vi "Health Status Screen 2.vi"() -> ()   [LabVIEW 2022 SP3]
panel:
  out "?":bool
  out "?":bool
  out "?":bool
  out "?":bool
  out "?":bool
  in  "Button":bool
  # "HEALTH STATUS"
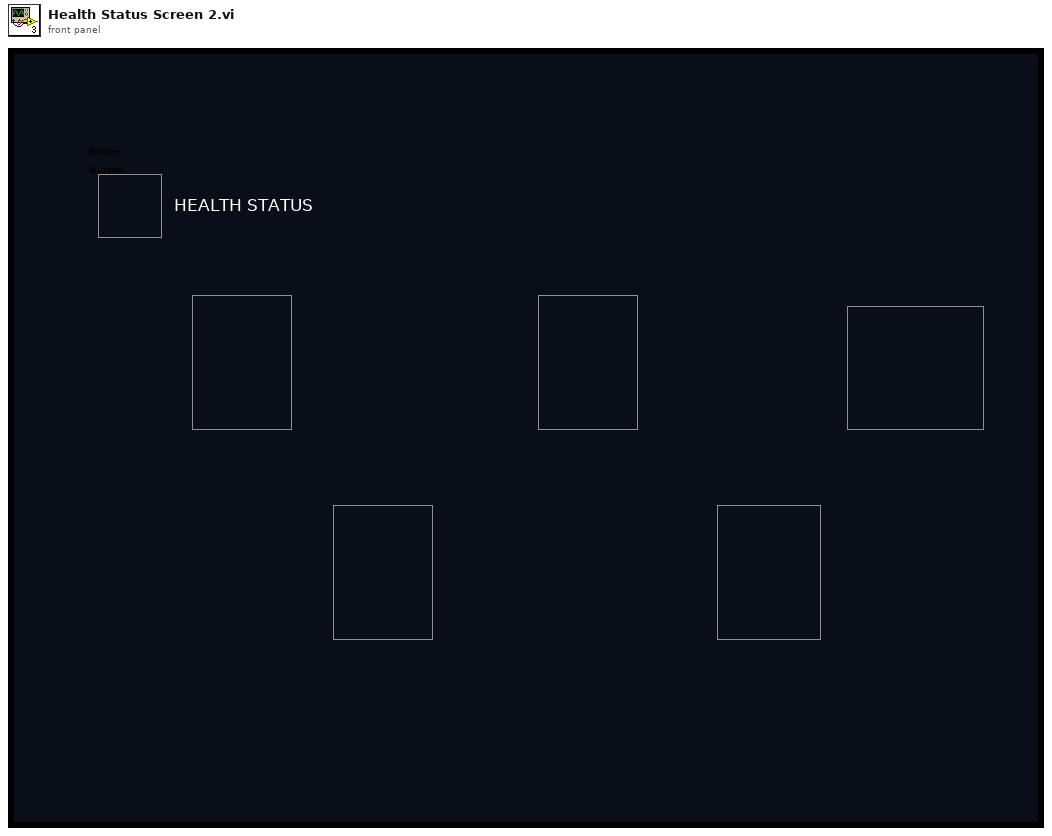
[diagram p1: front panel]
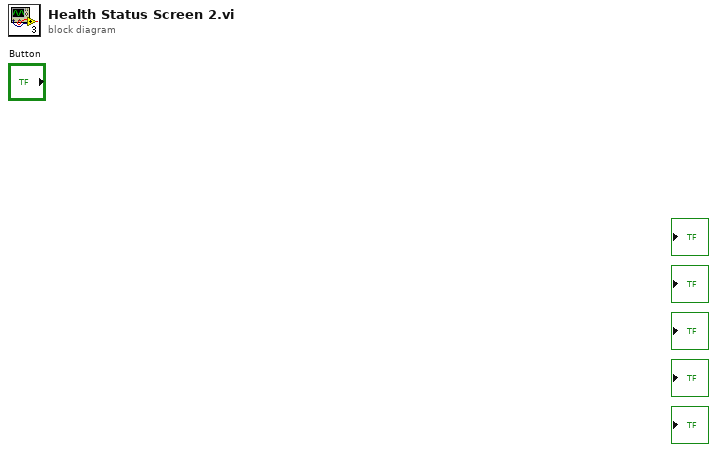
[diagram p0: block diagram]
diagram:
